vi "TWM Client Measure and Get Result.vi"(0 "handle":i32, 1 "end of packet key":string="TWM:command:EndOfPacket", 3 "timeout [s] (10s)":dbl=30.0, 5 "meas root path (last)":path, 7 "quantity names (all)":string[](array[string]), 9 "stop ref (none)":refnum<vi>, 11 "error in":errorcluster, 12 "qwtb maxdim (scalar)":T3 caption="Max. shown dimension (scalar)", 14 "phase ref channel tag (none)":string) -> (4 "handle out":i32, 6 "data":T2[][](array[typedef]), 8 "stoped?":bool, 10 "quantities":T1, 15 "error out":errorcluster)   [LabVIEW 2020, in "TWM Client.lvlib"]
doc: "TWM client top level function: Start measurement, wait for completion, Get result.\n\nSet reasonable timeout for the TWM sampling and processing. Wire in the the 'stop' reference to allow termination of the TWM task."
uses:
  TWM Client.lvlib
  TWM Client Result Max Dim.ctl
  TWM Client Quantity Record.ctl
  TWM Client Result Info.ctl
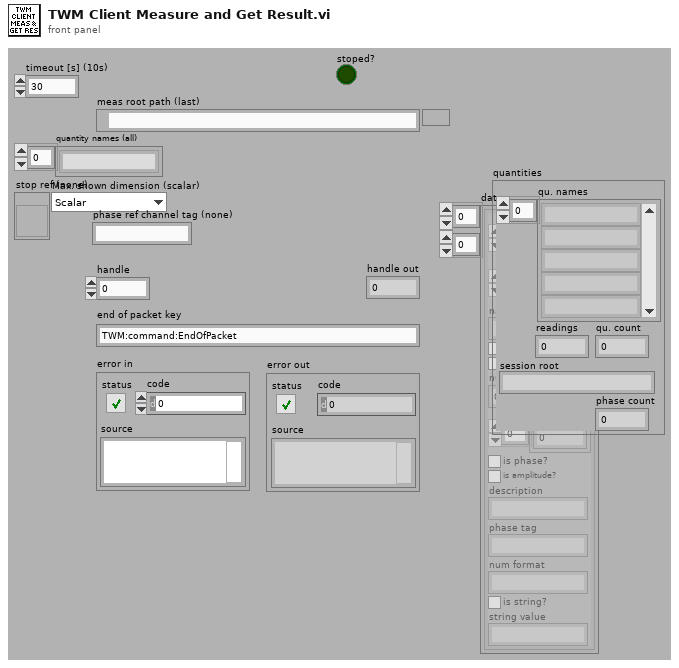
[diagram p1: front panel]
types:
  T1 = typedef "TWM Client.lvlib/TWM Client Result Info.ctl" = cluster{"qu. names":string[], "readings":i32, "qu. count":i32, "session root":string, "phase count":i32}
  T2 = typedef "TWM Client.lvlib/TWM Client Quantity Record.ctl" = cluster{"val":dbl[], "unc":dbl[], "name":string, "is valid?":bool, "has unc?":bool, "numel":i32, "ua":dbl[], "is phase?":bool, "is amplitude?":bool, "description":string, "phase tag":string, "num format":string, "is string?":bool, "string value":string}
  T3 = typedef "TWM Client.lvlib/TWM Client Result Max Dim.ctl" = enum16{"Scalar", "Vector", "Matrix"}
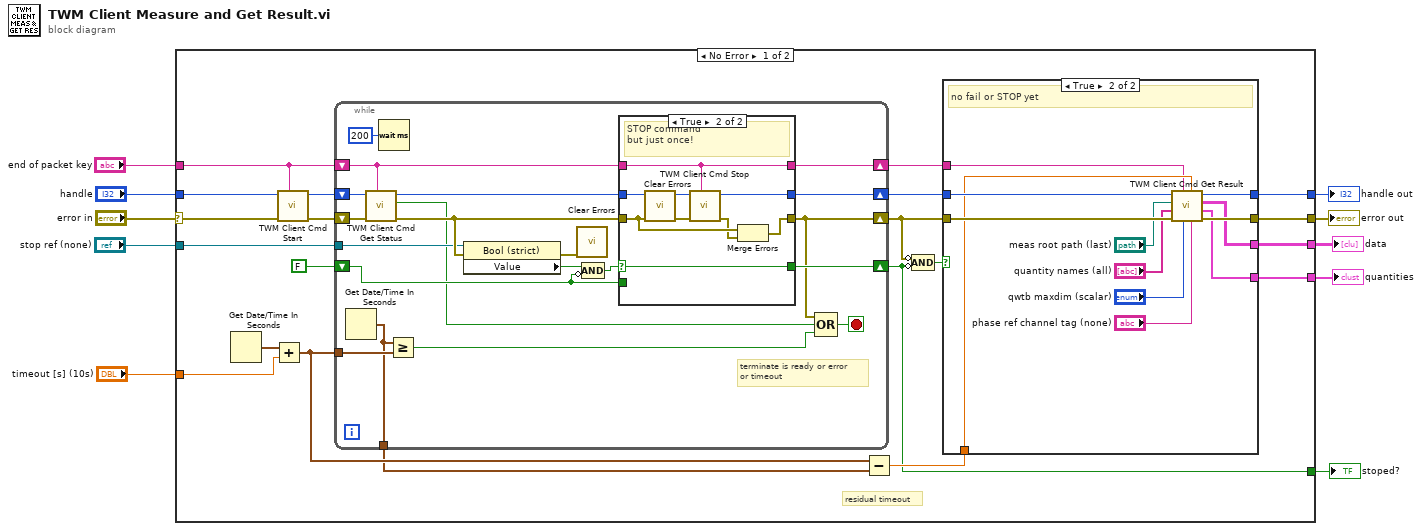
[diagram p0: block diagram]
diagram:
  n1 = case shown="No Error" "error in" {
    selector: "error in" -> [w12 w79]
    tunnel: "handle" -> [w31 w78]
    tunnel: "stop ref (none)" -> [w28 _]
    tunnel: "timeout [s] (10s)" -> [w26 _]
    tunnel: "end of packet key" -> [w25 _]
    tunnel: [w18 w78] -> w6
    tunnel: [w17 w79] -> w5
    tunnel: [w14 _] -> w4
    tunnel: [w13 _] -> w3
    tunnel: [w11 _] -> w1
    frame No Error {
      # "residual timeout"
      n2 = Get Date/Time In Seconds() -> (seconds since 1Jan1904=w24:timestamp)
      n3 = Add(x=w24, y=w26) -> (x+y=w23:timestamp)
      n4 = call "TWM Client Cmd Start.vi"("end of packet key"=w25, "error in"=w12, "handle"=w31) -> ("error out"=w30:errorcluster, "handle out"=w29:i32)  [unwired: 7 in]
      n5 = while {
        shift-right: [w59] -> w19
        shift-left: w29 -> [w65]
        shift-right: [w52] -> w20
        shift-left: w30 -> [w64]
        tunnel: w28 -> [w61]
        shift-right: [w58] -> w11
        shift-left: FALSE -> [w55]
        tunnel: w23 -> [w54]
        tunnel: [w47] -> w22
        shift-right: [w46] -> w15
        shift-left: w25 -> [w53]
        stop <- w49 stop-if-true
        # "terminate is ready or error\nor timeout"
        n6 = Get Date/Time In Seconds() -> (seconds since 1Jan1904=w47:timestamp)
        n7 = call "TWM Client Cmd Get Status.vi"("end of packet key"=w53, "error in"=w64, "handle"=w65) -> ("error out"=w63:errorcluster, "ready?"=w51:bool, "handle out"=w60:i32)  [unwired: 4 in, 2 out]
        n8 = Wait (ms)(milliseconds to wait=u32 200) -> ()  [unwired: 1 out]
        n9 = Greater Or Equal?(x=w47, y=w54) -> (x >= y?=w50:bool)
        n10 = property class="Bool (strict)"(reference=w61, error in=w63) -> (error out=w62:errorcluster, "Value"=w57:bool)  [unwired: 1 out]
        n11 = call <vilib>:"Clear Errors.vi"("error in (no error)"=w62) -> ()  [unwired: 5 in, 2 out]
        n12 = Compound Arithmetic op=AND(w57, invert w55) -> (w56:bool)
        n13 = case shown="True" w56 {
          selector: w56 -> [_ w71]
          tunnel: w63 -> [w69 w74]
          tunnel: w60 -> [w68 w76]
          tunnel: [w68 w75] -> w59
          tunnel: [w69 w72] -> w52
          tunnel: [w67 w71] -> w58
          tunnel: w55 -> [w67 _]
          tunnel: w53 -> [w66 w70]
          tunnel: [w66 w70] -> w46
          frame False {
          }
          frame True {
            # "STOP command\nbut just once!"
            n14 = call <vilib>:"Clear Errors.vi"("error in (no error)"=w74) -> ("error out"=w77:errorcluster)  [unwired: 5 in, 1 out]
            n15 = call "TWM Client Cmd Stop.vi"("end of packet key"=w70, "error in"=w77, "handle"=w76) -> ("error out"=w73:errorcluster, "handle out"=w75:i32)  [unwired: 7 in]
            n16 = Merge Errors(w74, w73) -> (w72:errorcluster)
          }
        }
        n17 = Compound Arithmetic op=OR(w52, w51, w50) -> (w49:bool)
      }
      n18 = Subtract(x=w23, y=w22) -> (x-y=w16:dbl)
      n19 = Compound Arithmetic op=AND(invert w20, invert w11) -> (w21:bool)
      n20 = case shown="True" w21 {
        tunnel: w20 -> [w33 w45]
        tunnel: w19 -> [w32 w44]
        tunnel: [w33 w43] -> w17
        tunnel: [w32 w42] -> w18
        tunnel: w16 -> [_ w38]
        tunnel: w15 -> [_ w37]
        tunnel: [_ w36] -> w14
        tunnel: [_ w35] -> w13
        frame False {
          # "STOP or error"
        }
        frame True {
          # "no fail or STOP yet"
          n21 = call "TWM Client Cmd Get Result.vi"("phase ref channel tag (none)"="phase ref channel tag (none)", "timeout [s] (10s)"=w38, "qwtb maxdim (scalar)"="qwtb maxdim (scalar)", "end of packet key"=w37, "error in"=w45, "quantity names (all)"="quantity names (all)", "meas root path (last)"="meas root path (last)", "handle"=w44) -> ("error out"=w43:errorcluster, "result info"=w35:T1, "result data"=w36:T2[][], "handle out"=w42:i32)
        }
      }
    }
    frame Error {
    }
  }
  "error out" <- w5
  "handle out" <- w6
  "data" <- w4
  "quantities" <- w3
  "stoped?" <- w1
